vi "Load App.vi"(6 "Open Actor Core front panel? (F)":bool, 8 "Error In":errorcluster, 11 "Status Notifier":refnum<notifier>) -> (0 "Error Out":errorcluster)   [LabVIEW 2015, in "Cap Bank Server.lvclass"]
uses:
  Cap Bank Server.lvclass
  <vilib>/ActorFramework/Actor/Actor.lvclass
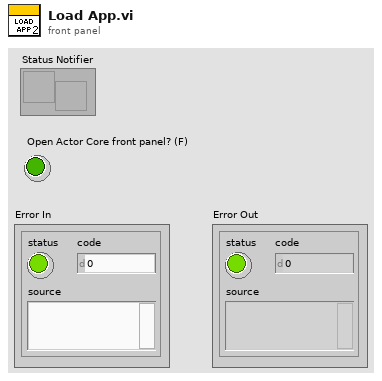
[diagram p1: front panel]
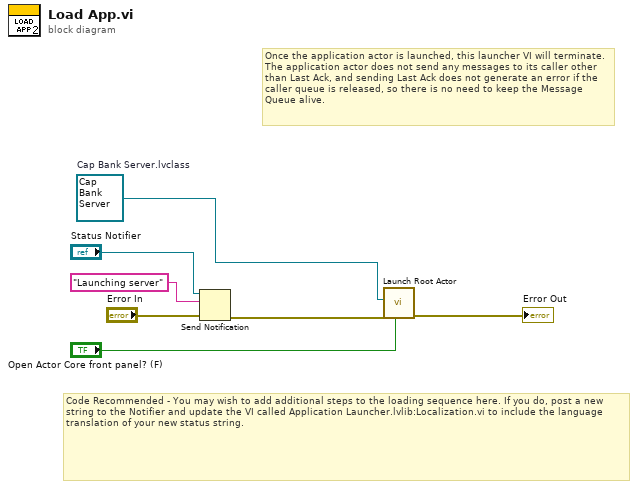
[diagram p0: block diagram]
diagram:
  w7 = refnum<class "Cap Bank Server.lvclass"> refnum  # Cap Bank Server.lvclass
  # "Code Recommended - You may wish to add additional steps to the loading sequence here. If you do, post a new string to the Notifier and update the VI called Application Launcher.lvlib:Localization.vi to include the language translation of your new status string."
  # "Once the application actor is launched, this launcher VI will terminate. The application actor does not send any messages to its caller other than Last Ack, and sending Last Ack does not generate an error if the caller queue is released, so there is no need to keep the Message Queue alive."
  n1 = Send Notification(notification="Launching server", notifier="Status Notifier", error in (no error)="Error In") -> (error out=w2:errorcluster)  [unwired: 1 out]
  n2 = call <vilib>:"Launch Root Actor.vi"("Open Actor Core front panel? (F)"="Open Actor Core front panel? (F)", "error in (no error)"=w2, "Actor"=w7) -> ("error out"=→"Error Out":errorcluster)  [unwired: 7 in, 1 out]
